vi "Read Ico File.vi"(8 "error in (no error)":errorcluster, 10 "Image Index":i32, 11 "Ico File":path=path "C:/Code/SVN/LabVIEW_Sandbox/Icon Extractor/Samsung SDI EOL Icon.ico") -> (0 "error out":errorcluster, 2 "Number Of Images":u16, 3 "Byte Array":u8[](array[numeric]) format="%.0x")   [LabVIEW 2019]
doc: "This VI will open an ICO file, and return an array of bytes that is the image selected by Image Index.\n\n-----\nBrian Hoover (Hooovahh)"
panel:
  out "Offset":u32
  out "Size":u32
  out "Bits Per Pixel":u16
  out "Color Planes":u16
  out "Colors In Color Palette":u8
  out "Height":u8
  out "Width":u8
  out "Image Type":u16
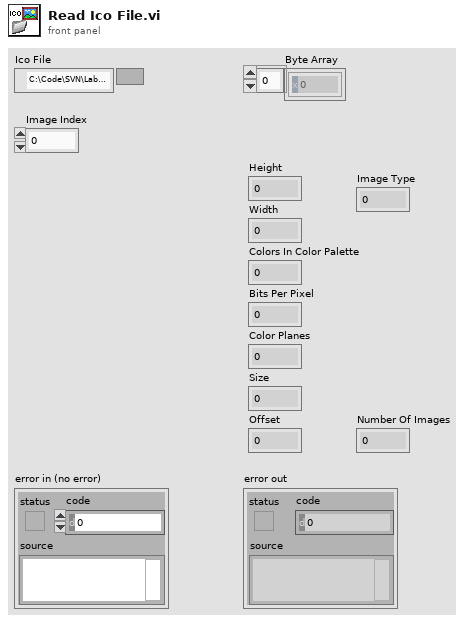
[diagram p1: front panel]
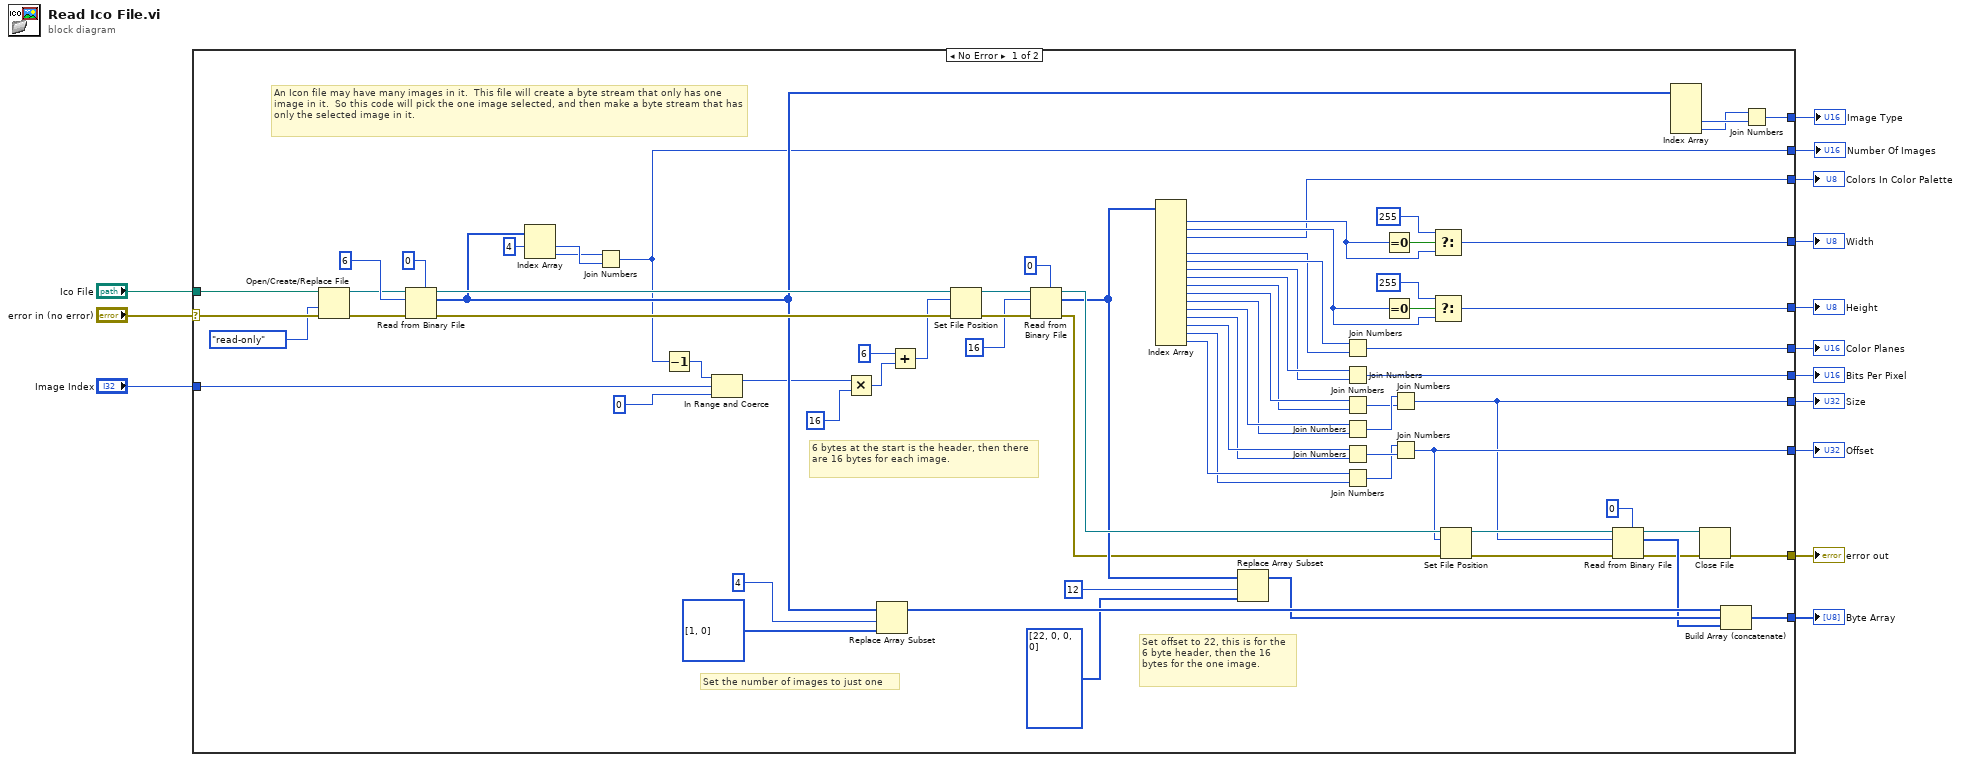
[diagram p0: block diagram]
diagram:
  n1 = case shown="No Error" "error in (no error)" {
    selector: "error in (no error)" -> [w32 w90]
    tunnel: "Ico File" -> [w26 _]
    tunnel: [w85 _] -> w13
    tunnel: [w16 _] -> w12
    tunnel: [w80 _] -> w11
    tunnel: [w74 _] -> w10
    tunnel: [w73 _] -> w9
    tunnel: [w69 _] -> w8
    tunnel: [w64 _] -> w7
    tunnel: [w63 _] -> w6
    tunnel: [w49 _] -> w5
    tunnel: [w45 _] -> w4
    tunnel: "Image Index" -> [w18 _]
    tunnel: [w29 w90] -> w1
    frame No Error {
      # "6 bytes at the start is the header, then there are 16 bytes for each image."
      # "Set the number of images to just one"
      # "An Icon file may have many images in it.  This file will create a byte stream that only has one image in it.  So this code will pick the one image selected, and then make a byte stream that has only the selected image in it."
      # "Set offset to 22, this is for the 6 byte header, then the 16 bytes for the one image."
      n2 = Open/Create/Replace File(file path (use dialog)=w26, error in=w32, access (0:read/write)=enum16{"read/write", "read-only", "write-only"}."read-only") -> (refnum out=w25:refnum<file>, error out=w27:errorcluster)  [unwired: 3 in, 1 out]
      n3 = Read from Binary File(5:u8 0, 8:w27, 10:6 ("count (1)"), 11:w25) -> (0:w84:errorcluster, 2:w20:u8[], 3:w37:refnum<file>)  [unwired: 2 in, 1 out]
      n4 = Index Array(array=w20, index #1=4 ("index")) -> (element #1=w22:u8, element #2=w21:u8)  [unwired: 1 in]
      n5 = Join Numbers(hi=w21, lo=w22) -> ((hi.lo)=w16:u16)
      n6 = Decrement(x=w16) -> (x-1=w15:u16)
      n7 = In Range and Coerce(upper limit=w15, x=w18, lower limit=0) -> (coerced(x)=w17:i32)  [unwired: 1 out]
      n8 = Multiply(x=w17, y=16) -> (x*y=w40:i32)
      n9 = Replace Array Subset(array=w20, new element=u8[] [1, 0], index=4) -> (w83:u8[])
      n10 = Add(x=6, y=w40) -> (x+y=w34:i32)
      n11 = Set File Position(offset (in bytes) (0)=w34, refnum=w37, error in=w84) -> (refnum out=w36:refnum<file>, error out=w38:errorcluster)  [unwired: 1 in]
      n12 = Read from Binary File(5:u8 0, 8:w38, 10:16 ("count (1)"), 11:w36) -> (0:w30:errorcluster, 2:w44:u8[], 3:w50:refnum<file>)  [unwired: 2 in, 1 out]
      n13 = Index Array(array=w44) -> (element #1=w71:u8, element #2=w70:u8, element #3=w69:u8, element #5=w67:u8, element #6=w68:u8, element #7=w65:u8, element #8=w66:u8, element #9=w61:u8, element #10=w62:u8, element #11=w59:u8, element #12=w60:u8, element #13=w53:u8, element #14=w54:u8, element #15=w51:u8, element #16=w52:u8)  [unwired: 16 in, 1 out]
      n14 = Replace Array Subset(array=w44, new element=u8[] [22, 0, 0, 0], index=12) -> (w43:u8[])
      n15 = Join Numbers(hi=w68, lo=w67) -> ((hi.lo)=w64:u16)
      n16 = Join Numbers(hi=w66, lo=w65) -> ((hi.lo)=w63:u16)
      n17 = Join Numbers(hi=w62, lo=w61) -> ((hi.lo)=w57:u16)
      n18 = Join Numbers(hi=w60, lo=w59) -> ((hi.lo)=w58:u16)
      n19 = Join Numbers(hi=w54, lo=w53) -> ((hi.lo)=w56:u16)
      n20 = Join Numbers(hi=w52, lo=w51) -> ((hi.lo)=w55:u16)
      n21 = Equal To 0?(x=w71) -> (x = 0?=w78:bool)
      n22 = Equal To 0?(x=w70) -> (x = 0?=w75:bool)
      n23 = Join Numbers(hi=w58, lo=w57) -> ((hi.lo)=w45:u32)
      n24 = Join Numbers(hi=w55, lo=w56) -> ((hi.lo)=w49:u32)
      n25 = Select(t=u8 255, s=w78, f=w71) -> (s? t:f=w74:u8)
      n26 = Select(t=u8 255, s=w75, f=w70) -> (s? t:f=w73:u8)
      n27 = Set File Position(offset (in bytes) (0)=w49, refnum=w50, error in=w30) -> (refnum out=w47:refnum<file>, error out=w46:errorcluster)  [unwired: 1 in]
      n28 = Read from Binary File(5:u8 0, 8:w46, 10:w45, 11:w47) -> (0:w31:errorcluster, 2:w41:u8[], 3:w28:refnum<file>)  [unwired: 2 in, 1 out]
      n29 = Index Array(array=w20) -> (element #3=w87:u8, element #4=w86:u8)  [unwired: 4 in, 2 out]
      n30 = Close File(refnum=w28, error in=w31) -> (error out=w29:errorcluster)  [unwired: 1 out]
      n31 = Build Array (concatenate)(w83, w43, w41) -> (w80:u8[])
      n32 = Join Numbers(hi=w86, lo=w87) -> ((hi.lo)=w85:u16)
    }
    frame Error {
    }
  }
  "Number Of Images" <- w12
  "Image Type" <- w13
  "Byte Array" <- w11
  "Width" <- w10
  "Height" <- w9
  "Colors In Color Palette" <- w8
  "Color Planes" <- w7
  "Bits Per Pixel" <- w6
  "Size" <- w4
  "Offset" <- w5
  "error out" <- w1
